vi "Destroy.vi"(8 "error in (no error)":errorcluster, 11 ".NET Process in":refnum<class "SystemProcessManager.lvclass">) -> (0 "error out":errorcluster, 3 ".NET Process out":refnum<class "SystemProcessManager.lvclass">)   [LabVIEW 2019, in "SystemProcessManager.lvclass"]
uses:
  SystemProcessManager.lvclass
  SystemProcessManager.lvclass/SystemProcessManager.ctl
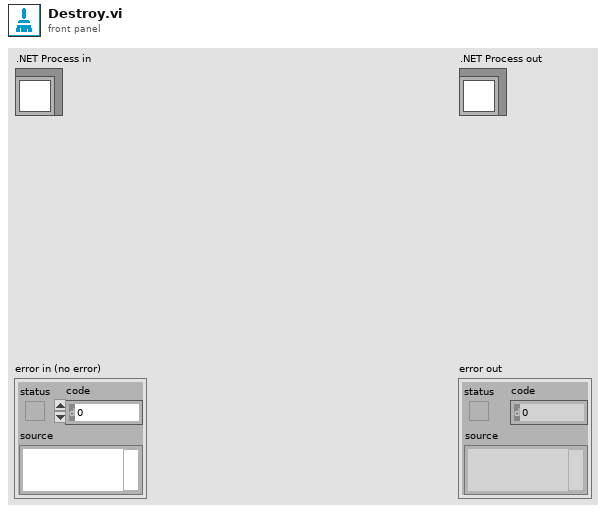
[diagram p1: front panel]
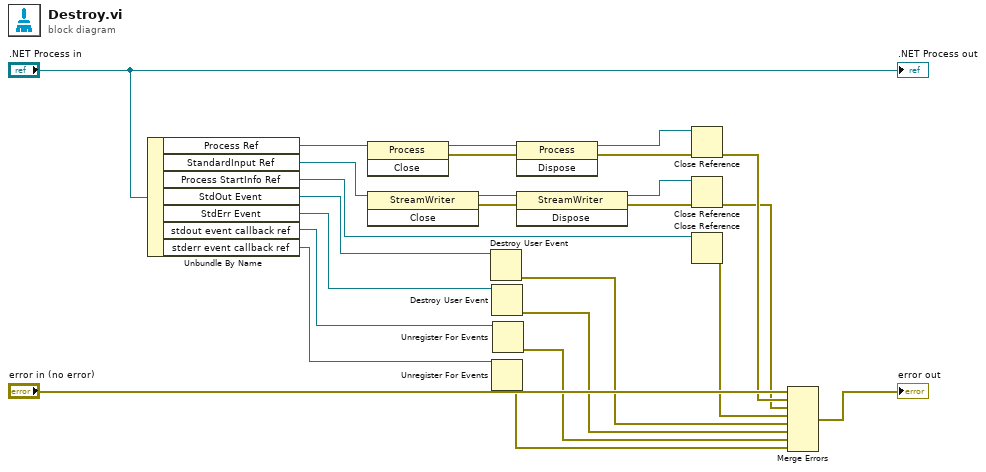
[diagram p0: block diagram]
diagram:
  n1 = Unbundle By Name(".NET Process in") -> ("Process Ref"=w12:refnum<k24>, "StandardInput Ref"=w11:refnum<k24>, "Process StartInfo Ref"=w10:refnum<k24>, "StdOut Event"=w8:refnum<user-event>, "StdErr Event"=w7:refnum<user-event>, "stdout event callback ref"=w4:refnum<k27>, "stderr event callback ref"=w3:refnum<k27>)
  n2 = invoke class="Process" method="Close"(reference=w12) -> (reference out=w18:refnum<k24>, error out=w17:errorcluster)  [unwired: 2 in, 1 out]
  n3 = invoke class="StreamWriter" method="Close"(reference=w11) -> (reference out=w22:refnum<k24>, error out=w21:errorcluster)  [unwired: 2 in, 1 out]
  n4 = Destroy User Event(user event=w8) -> (error out=w6:errorcluster)  [unwired: 1 in]
  n5 = Destroy User Event(user event=w7) -> (error out=w5:errorcluster)  [unwired: 1 in]
  n6 = Unregister For Events(event registration refnum=w3) -> (error out=w1:errorcluster)  [unwired: 1 in]
  n7 = Unregister For Events(event registration refnum=w4) -> (error out=w2:errorcluster)  [unwired: 1 in]
  n8 = invoke class="Process" method="Dispose"(reference=w18, error in=w17) -> (reference out=w15:refnum<k24>, error out=w16:errorcluster)  [unwired: 1 in, 1 out]
  n9 = invoke class="StreamWriter" method="Dispose"(reference=w22, error in=w21) -> (reference out=w19:refnum<k24>, error out=w20:errorcluster)  [unwired: 1 in, 1 out]
  n10 = Close Reference(reference=w15, error in (no error)=w16) -> (error out=w14:errorcluster)
  n11 = Close Reference(reference=w19, error in (no error)=w20) -> (error out=w13:errorcluster)
  n12 = Close Reference(reference=w10) -> (error out=w9:errorcluster)  [unwired: 1 in]
  n13 = Merge Errors("error in (no error)", w14, w13, w9, w6, w5, w2, w1) -> (→"error out":errorcluster)
  ".NET Process out" <- ".NET Process in"
